vi "Database FGV.vi"(8 "error in (no error)":errorcluster, 9 "Database Records In":T1[](array[typedef]), 10 "Database Record":T1, 11 "Database Action":T2) -> (0 "error out":errorcluster, 1 "Database Records":T1[](array[typedef]), 3 "Timing Array":i16[](array[numeric]))   [LabVIEW 2012, in "Architecture.lvlib" / "Database.lvclass"]
uses:
  Database.lvclass
  <vilib>/Utility/xml.llb/Read From XML File(string).vi
  Database Action.ctl
  Database Record.ctl
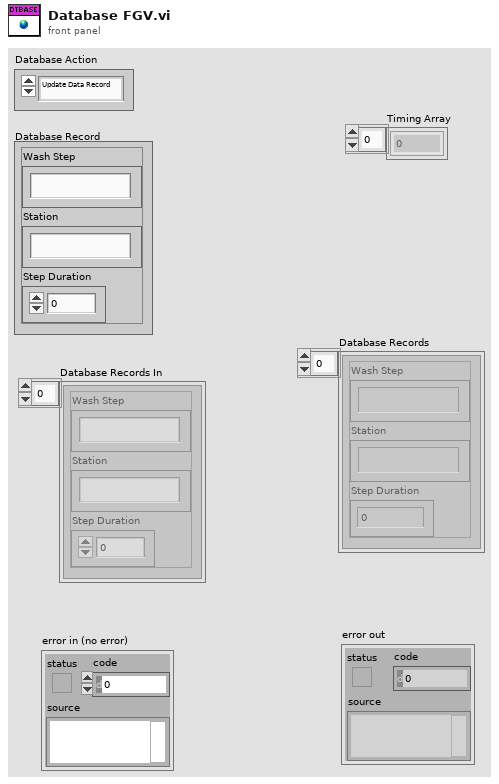
[diagram p1: front panel]
types:
  T1 = typedef "Architecture.lvlib/Database.lvclass/Database Record.ctl" = cluster{"Wash Step":string, "Station":string, "Step Duration":i16}
  T2 = typedef "Architecture.lvlib/Database.lvclass/Database Action.ctl" = enum16{"Update Data Record", "Insert New Data Record", "Query Timing Data", "Read Records", "Initialize"}
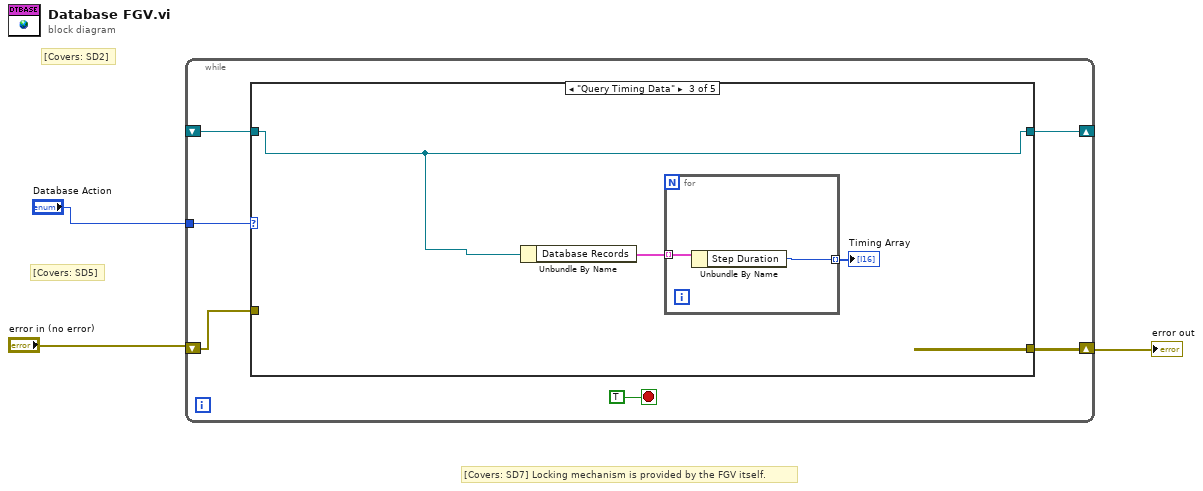
[diagram p0: block diagram]
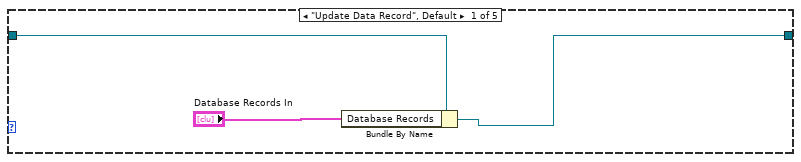
[diagram p2: hidden frame]
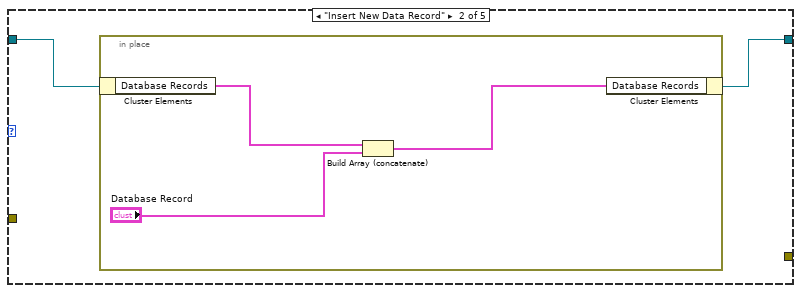
[diagram p3: hidden frame]
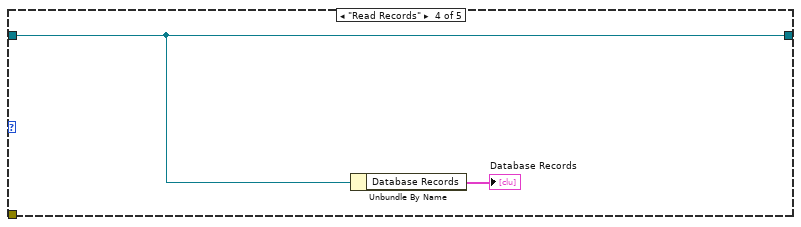
[diagram p4: hidden frame]
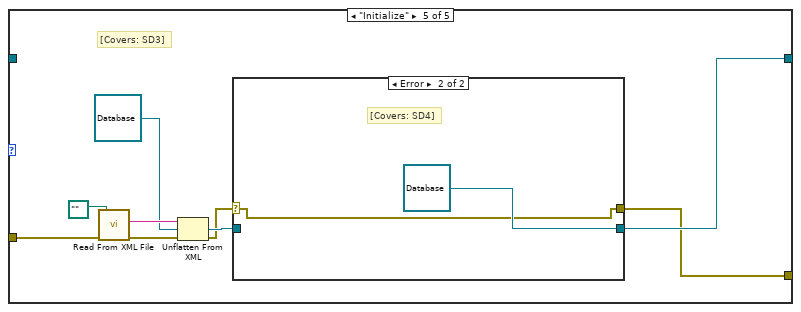
[diagram p5: hidden frame]
diagram:
  # "[Covers: SD7] Locking mechanism is provided by the FGV itself."
  # "[Covers: SD5]"
  # "[Covers: SD2]"
  n1 = while {
    shift-right: [w9] -> _
    shift-left: _ -> [w4]
    tunnel: "Database Action" -> [w7]
    shift-right: [w5] -> w3
    shift-left: "error in (no error)" -> [w6]
    stop <- TRUE stop-if-true
    n2 = case shown="\"Query Timing Data\"" w7 {
      tunnel: [w11 w13 w18 w23 w29] -> w9
      tunnel: w6 -> [_ _ _ _ w27]
      tunnel: [_ _ _ _ w25] -> w5
      tunnel: w4 -> [w12 w14 w18 w23 _]
      frame "Update Data Record", Default {
        n3 = Bundle By Name(cluster=w12, "Database Records"="Database Records In") -> (w11:refnum<class "Database.lvclass">)
      }
      frame "Insert New Data Record" {
        n4 = in-place {
          n5 = in-place-cluster #1(w14) -> ("Database Records"=w17:T1[])
          n6 = Build Array (concatenate)(w17, "Database Record") -> (w16:T1[])
          n7 = in-place-cluster #1("Database Records"=w16) -> (w13:refnum<class "Database.lvclass">)
        }
      }
      frame "Query Timing Data" {
        n8 = Unbundle By Name(w18) -> ("Database Records"=w20:T1[])
        n9 = for {
          tunnel: w20 -> [w22] mode=indexing
          tunnel: [w21] -> w19 mode=indexing
          n10 = Unbundle By Name(w22) -> ("Step Duration"=w21:i16)
        }
        "Timing Array" <- w19
      }
      frame "Read Records" {
        n11 = Unbundle By Name(w23) -> ("Database Records"=→"Database Records":T1[])
      }
      frame "Initialize" {
        # "[Covers: SD3]"
        n12 = call-poly <vilib>:"Read From XML File.vi"("error in (no error)"=w27, "XML File Path"=path "") -> ("error out"=w32:errorcluster, "XML Elements"=w31:string)  [unwired: 7 in, 1 out]
        n13 = Unflatten From XML(xml string=w31, type=refnum<class "Database.lvclass"> refnum ("Database in"), error in (no error)=w32) -> (value=w28:refnum<class "Database.lvclass">, error out=w26:errorcluster)
        n14 = case shown="Error" w26 {
          selector: w26 -> [w34 w36]
          tunnel: [w35 refnum<class "Database.lvclass"> refnum ("Database in")] -> w29
          tunnel: w28 -> [w35 _]
          tunnel: [w34 w36] -> w25
          frame No Error {
          }
          frame Error {
            # "[Covers: SD4]"
          }
        }
      }
    }
  }
  "error out" <- w3
